vi "GetFileCreationDate(SubVI).vi"(6 "Error In":errorcluster, 9 "File Path":path) -> (0 "Error Out":errorcluster, 3 "File Created Date (UTC)":timestamp)   [LabVIEW 2018, in "MainFrameLib.lvlib"]
uses:
  MainFrameLib.lvlib
  kernel32.dll
panel:
  in  "date time rec":T1
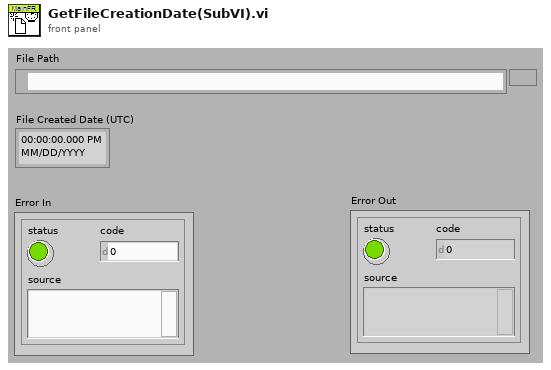
[diagram p1: front panel]
types:
  T1 = cluster{"fractional second":dbl, "second":i32, "minute":i32, "hour":i32, "day of month":i32, "month":i32, "year":i32, "day of week":i32, "day of year":i32, "DST":i32}
  T2 = cluster{"wYear":u16, "wMonth":u16, "wDayOfWeek":u16, "wDay":u16, "wHour":u16, "wMinute":u16, "wSeconds":u16, "wMilliseconds":u16}
  T3 = cluster{"dwFileAttributes":i32, "ftCreationTime":cluster{"dwLowDateTime":i32, "dwHighDateTime":i32}, "ftLastAccessTime":cluster{"dwLowDateTime":i32, "dwHighDateTime":i32}, "ftLastWrittenTime":cluster{"dwLowDateTime":i32, "dwHighDateTime":i32}, "nFileSizeHigh":i32, "nFileSizeLow":i32}
  T4 = cluster{"dwLowDateTime":i32, "dwHighDateTime":i32}
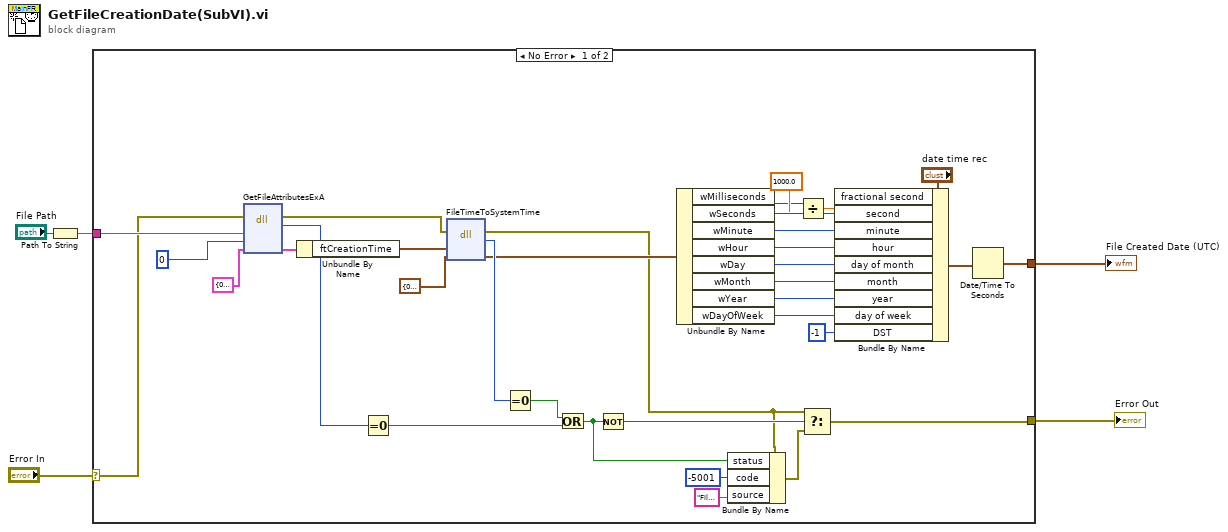
[diagram p0: block diagram]
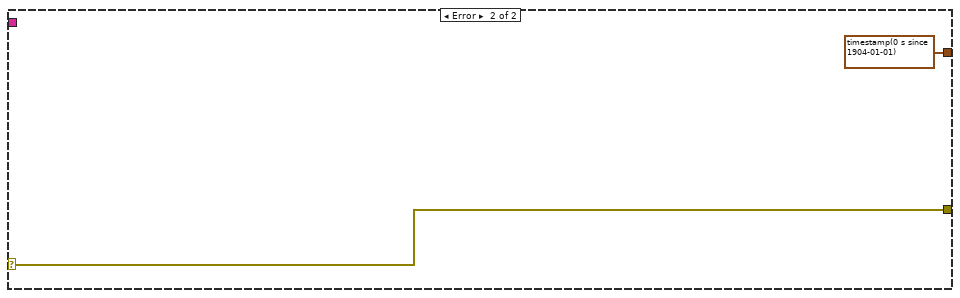
[diagram p2: hidden frame]
diagram:
  n1 = Path To String(path="File Path") -> (string=w4:string)
  n2 = case shown="No Error" "Error In" {
    selector: "Error In" -> [w16 w41]
    tunnel: w4 -> [w39 _]
    tunnel: [w23 timestamp(0 s since 1904-01-01) ("time stamp")] -> w3
    tunnel: [w6 w41] -> w1
    frame No Error {
      n3 = dll-call lib="kernel32.dll" fn="GetFileAttributesExA"(error in=w16, "lpFileName"=w39, "fInfoLevelID"=0, "output param"=T3 {"dwFileAttributes"=0, "ftCreationTime"={"dwLowDateTime"=0, "dwHighDateTime"=0}, "ftLastAccessTime"={"dwLowDateTime"=0, "dwHighDateTime"=0}, "ftLastWrittenTime"={"dwLowDateTime"=0, "dwHighDateTime"=0}, "nFileSizeHigh"=0, "nFileSizeLow"=0}) -> (error out=w15:errorcluster, w33:i32, "output param"=w36:T3)  [unwired: 4 in, 1 out]
      n4 = Unbundle By Name(w36) -> ("ftCreationTime"=w35:T4)
      n5 = Equal To 0?(x=w33) -> (x = 0?=w14:bool)
      n6 = dll-call lib="kernel32.dll" fn="FileTimeToSystemTime"(error in=w15, "ftCreationTime"=w35, "output param"=T2 {"wYear"=0, "wMonth"=0, "wDayOfWeek"=0, "wDay"=0, "wHour"=0, "wMinute"=0, "wSeconds"=0, "wMilliseconds"=0}) -> (error out=w11:errorcluster, w32:i32, "output param"=w31:T2)  [unwired: 3 in, 1 out]
      n7 = Equal To 0?(x=w32) -> (x = 0?=w13:bool)
      n8 = Or(x=w13, y=w14) -> (x .or. y?=w9:bool)
      n9 = Not(x=w9) -> (.not. x?=w12:bool)
      n10 = Unbundle By Name(w31) -> ("wMilliseconds"=w20:u16, "wSeconds"=w30:u16, "wMinute"=w29:u16, "wHour"=w28:u16, "wDay"=w27:u16, "wMonth"=w26:u16, "wYear"=w25:u16, "wDayOfWeek"=w24:u16)
      n11 = Bundle By Name(cluster=w11, "status"=w9, "code"=-5001, "source"="File error in GetFileCreationDate(SubVI): Check if the path to the file is correct or if thre is any file corruption") -> (w10:errorcluster)
      n12 = Divide(x=w20, y=1000.0) -> (x/y=w19:dbl)
      n13 = Select(t=w11, s=w12, f=w10) -> (s? t:f=w6:errorcluster)
      n14 = Bundle By Name(cluster="date time rec", "fractional second"=w19, "second"=w30, "minute"=w29, "hour"=w28, "day of month"=w27, "month"=w26, "year"=w25, "day of week"=w24, "DST"=-1) -> (w18:T1)
      n15 = Date/Time To Seconds(2:w18) -> (0:w23:timestamp)  [unwired: 1 in]
    }
    frame Error {
    }
  }
  "File Created Date (UTC)" <- w3
  "Error Out" <- w1
